vi "UDB_decode_line_1.1.vi"(0 "arrayIn":i32[](array[numeric])) -> (4 "streap":i32[](array[numeric]), 5 "value":i32[](array[numeric]), 6 "silica":bool, 7 "tdc1":bool, 8 "peak":bool, 9 "qdc3":bool, 10 "qdc1":bool, 11 "tdc4":bool, 12 "qdc2":bool, 13 "scaler":i32[](array[numeric]), 14 "peak":i32[](array[numeric]), 15 "qdc1(prof)":i32[](array[numeric]), 16 "qdc2(calo)":i32[](array[numeric]), 17 "tdc1":i32[](array[numeric]), 18 "qdc3":i32[](array[numeric]), 19 "tdc4":i32[](array[numeric]))   [LabVIEW 2014]
panel:
  out "size(s)":i32
  out "N_silica":dbl
  out "null":bool
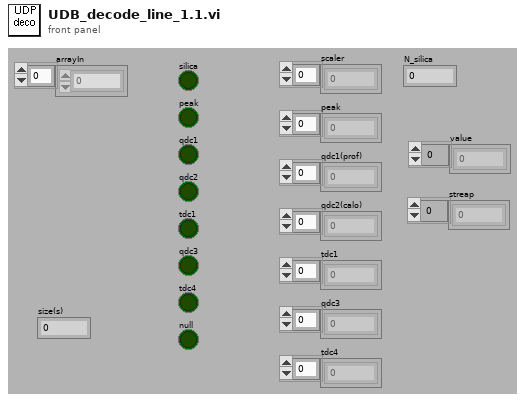
[diagram p1: front panel]
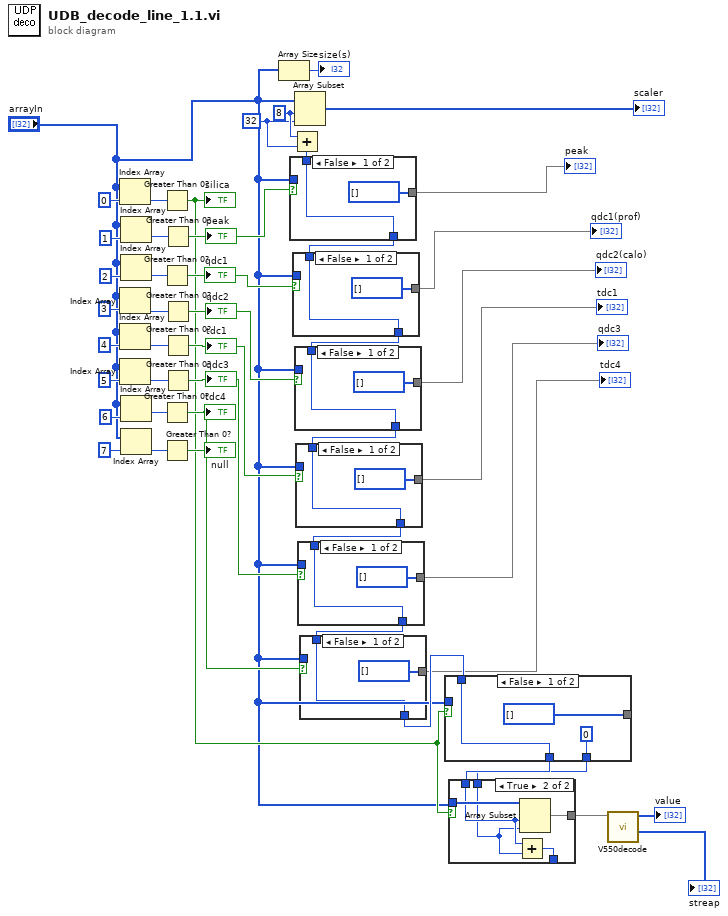
[diagram p0: block diagram]
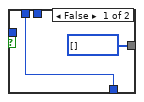
[diagram p2: hidden frame]
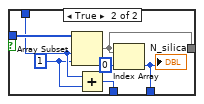
[diagram p3: hidden frame]
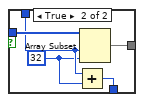
[diagram p4: hidden frame]
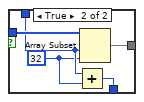
[diagram p5: hidden frame]
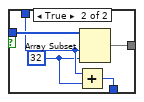
[diagram p6: hidden frame]
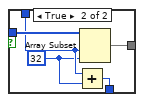
[diagram p7: hidden frame]
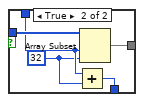
[diagram p8: hidden frame]
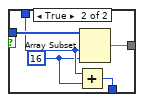
[diagram p9: hidden frame]
diagram:
  w27 = 32 ("length")
  w28 = 8 ("index")
  n1 = Index Array(array="arrayIn", index=0) -> (element=w38:i32)
  n2 = Index Array(array="arrayIn", index=3) -> (element=w35:i32)
  n3 = Index Array(array="arrayIn", index=4) -> (element=w34:i32)
  n4 = Index Array(array="arrayIn", index=5) -> (element=w33:i32)
  n5 = Index Array(array="arrayIn", index=1) -> (element=w37:i32)
  n6 = Index Array(array="arrayIn", index=2) -> (element=w36:i32)
  n7 = Index Array(array="arrayIn", index=6) -> (element=w32:i32)
  n8 = Index Array(array="arrayIn", index=7) -> (element=w31:i32)
  n9 = Greater Than 0?(x=w38) -> (x > 0?=w14:bool)
  "silica" <- w14
  n10 = Greater Than 0?(x=w36) -> (x > 0?=w25:bool)
  "qdc1" <- w25
  n11 = Greater Than 0?(x=w32) -> (x > 0?=w16:bool)
  "tdc4" <- w16
  n12 = Greater Than 0?(x=w31) -> (x > 0?=→"null":bool)
  n13 = Greater Than 0?(x=w37) -> (x > 0?=w29:bool)
  "peak" <- w29
  n14 = Greater Than 0?(x=w35) -> (x > 0?=w23:bool)
  "qdc2" <- w23
  n15 = Greater Than 0?(x=w34) -> (x > 0?=w21:bool)
  "tdc1" <- w21
  n16 = Greater Than 0?(x=w33) -> (x > 0?=w18:bool)
  "qdc3" <- w18
  n17 = Array Size(array="arrayIn") -> (size(s)=→"size(s)":i32)
  n18 = Add(x=w28, y=w27) -> (x+y=w26:i32)
  n19 = case shown="False" w29 {
    tunnel: "arrayIn" -> [_ w54]
    tunnel: w26 -> [w48 w53]
    tunnel: [i32[] [] w51] -> w12
    tunnel: [w48 w50] -> w24
    frame False {
    }
    frame True {
      w52 = 16 ("length")
      n20 = Add(x=w53, y=w52) -> (x+y=w50:i32)
      n21 = Array Subset(array=w54, index=w53, length=w52) -> (w51:i32[])
    }
  }
  "peak" <- w12
  n22 = case shown="False" w25 {
    tunnel: "arrayIn" -> [_ w61]
    tunnel: w24 -> [w55 w60]
    tunnel: [i32[] [] w58] -> w11
    tunnel: [w55 w57] -> w22
    frame False {
    }
    frame True {
      w59 = 32 ("length")
      n23 = Add(x=w60, y=w59) -> (x+y=w57:i32)
      n24 = Array Subset(array=w61, index=w60, length=w59) -> (w58:i32[])
    }
  }
  "qdc1(prof)" <- w11
  n25 = Array Subset(array="arrayIn", index=w28, length=w27) -> (→"scaler":i32[])
  n26 = case shown="False" w23 {
    tunnel: "arrayIn" -> [_ w68]
    tunnel: w22 -> [w62 w67]
    tunnel: [i32[] [] w65] -> w10
    tunnel: [w62 w64] -> w20
    frame False {
    }
    frame True {
      w66 = 32 ("length")
      n27 = Add(x=w67, y=w66) -> (x+y=w64:i32)
      n28 = Array Subset(array=w68, index=w67, length=w66) -> (w65:i32[])
    }
  }
  "qdc2(calo)" <- w10
  n29 = case shown="False" w21 {
    tunnel: "arrayIn" -> [_ w75]
    tunnel: w20 -> [w69 w74]
    tunnel: [i32[] [] w72] -> w9
    tunnel: [w69 w71] -> w19
    frame False {
    }
    frame True {
      w73 = 32 ("length")
      n30 = Add(x=w74, y=w73) -> (x+y=w71:i32)
      n31 = Array Subset(array=w75, index=w74, length=w73) -> (w72:i32[])
    }
  }
  "tdc1" <- w9
  n32 = case shown="False" w18 {
    tunnel: "arrayIn" -> [_ w82]
    tunnel: w19 -> [w76 w81]
    tunnel: [i32[] [] w79] -> w8
    tunnel: [w76 w78] -> w17
    frame False {
    }
    frame True {
      w80 = 32 ("length")
      n33 = Add(x=w81, y=w80) -> (x+y=w78:i32)
      n34 = Array Subset(array=w82, index=w81, length=w80) -> (w79:i32[])
    }
  }
  "qdc3" <- w8
  n35 = case shown="False" w16 {
    tunnel: "arrayIn" -> [_ w89]
    tunnel: w17 -> [w83 w88]
    tunnel: [i32[] [] w86] -> w7
    tunnel: [w83 w85] -> w15
    frame False {
    }
    frame True {
      w87 = 32 ("length")
      n36 = Add(x=w88, y=w87) -> (x+y=w85:i32)
      n37 = Array Subset(array=w89, index=w88, length=w87) -> (w86:i32[])
    }
  }
  "tdc4" <- w7
  n38 = case shown="False" w14 {
    tunnel: "arrayIn" -> [_ w99]
    tunnel: w15 -> [w91 w98]
    tunnel: [i32[] [] w94] -> _
    tunnel: [w91 w96] -> w13
    tunnel: [0 ("Numeric") w93] -> w6
    frame False {
    }
    frame True {
      w97 = 1 ("length")
      n39 = Array Subset(array=w99, index=w98, length=w97) -> (w94:i32[])
      n40 = Add(x=w98, y=w97) -> (x+y=w96:i32)
      n41 = Index Array(array=w94, index=0) -> (element=w93:i32)
      "N_silica" <- w93
    }
  }
  n42 = case shown="True" w14 {
    tunnel: "arrayIn" -> [_ w106]
    tunnel: w13 -> [w100 w105]
    tunnel: [i32[] [] w104] -> w5
    tunnel: [w100 w103] -> _
    tunnel: w6 -> [_ w102]
    frame False {
    }
    frame True {
      n43 = Add(x=w105, y=w102) -> (x+y=w103:i32)
      n44 = Array Subset(array=w106, index=w105, length=w102) -> (w104:i32[])
    }
  }
  n45 = call "V550decode.vi"("V550 data"=w5) -> ("streap"=→"streap":i32[], "value"=→"value":i32[])  [unwired: 5 in]
